vi "Start.vi"(7 "Timer ID":i32, 8 "error in (no error)":errorcluster, 10 "Target Time (seconds)":dbl, 11 "Timer in":refnum<class "Timer.lvclass">) -> (0 "error out":errorcluster, 3 "Timer DVR":refnum<data-value>)   [LabVIEW 2018, in "Timer.lvclass"]
uses:
  Timer.lvclass
  Timer.lvclass/Timer.ctl
  Set Target Time Elapsed Event.vi
  GUI.vi
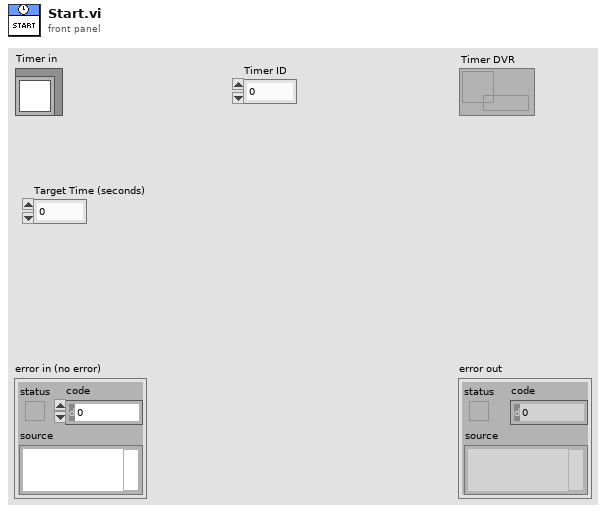
[diagram p1: front panel]
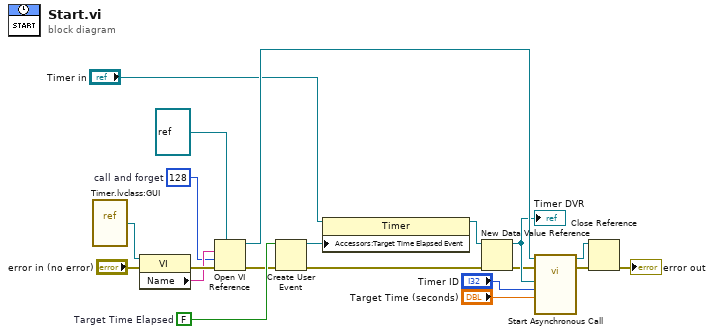
[diagram p0: block diagram]
diagram:
  w6 = FALSE  # Target Time Elapsed
  w13 = 128  # call and forget
  n1 = vi-ref "Timer.lvclass:GUI.vi"() -> (w18:refnum<vi>)
  n2 = property class="VI"(reference=w18, error in="error in (no error)") -> (error out=w20:errorcluster, "Name"=w19:string)  [unwired: 1 out]
  n3 = Open VI Reference(type specifier VI Refnum (for type only)=refnum<vi> refnum, vi path=w19, options=w13, error in (no error)=w20) -> (vi reference=w15:refnum<vi>, error out=w3:errorcluster)  [unwired: 2 in]
  n4 = Create User Event(user event datatype=w6, error in=w3) -> (user event=w4:refnum<user-event>, error out=w2:errorcluster)
  n5 = property class="Timer"(reference="Timer in", "Accessors:Target Time Elapsed Event"=w4) -> (reference out=w5:refnum<class "Timer.lvclass">)  [unwired: 1 in, 1 out]
  n6 = New Data Value Reference(data value=w5, error in=w2) -> (data value reference=w10:refnum<data-value>, error out=w7:errorcluster)
  "Timer DVR" <- w10
  n7 = call-by-ref "Start Asynchronous Call"(reference=w15, error in=w7, "Target Time (seconds)"="Target Time (seconds)", "Timer ID"="Timer ID", "Timer DVR"=w10) -> (reference out=w17:refnum<vi>, error out=w16:errorcluster)  [unwired: 9 in]
  n8 = Close Reference(reference=w17, error in (no error)=w16) -> (error out=→"error out":errorcluster)
